vi "ProcessName.vi"() -> (1 "ProcessName":string)   [LabVIEW 2017, in "McsaStartupAnalysis.lvlib"]
uses:
  <vilib>/addons/InsightCM/Devices/Shared/Mcsa/McsaStartupAnalysis/McsaStartupAnalysis.lvlib
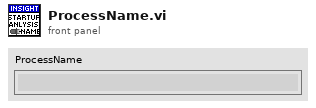
[diagram p1: front panel]
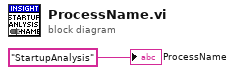
[diagram p0: block diagram]
diagram:
  "ProcessName" <- "StartupAnalysis" ("ProcessName")
